vi "Simulation Angle Step (SubVI).vi"(6 "n":dbl, 7 "N (Rot)":u32, 8 "error in (no error)":errorcluster, 10 "Final Angle":dbl, 11 "VISA Refnum in":refnum<visa-resource-name>) -> (0 "error out":errorcluster, 2 "Next Angle":dbl, 3 "VISA Refnum out":refnum<visa-resource-name>, 4 "Angle Time Step (ms)":dbl, 5 "Rotation Complete?":bool)   [LabVIEW 2012]
uses:
  Stage Global.vi
  Rotation Mount Global.vi
panel:
  # "**For steps of the form degrees = a(x-xi)^n"
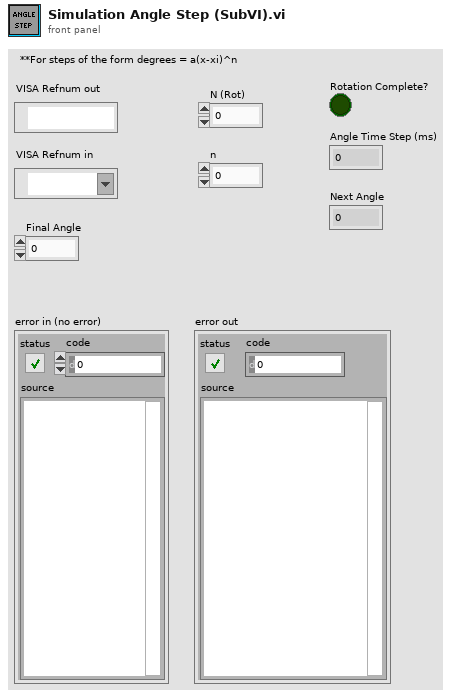
[diagram p1: front panel]
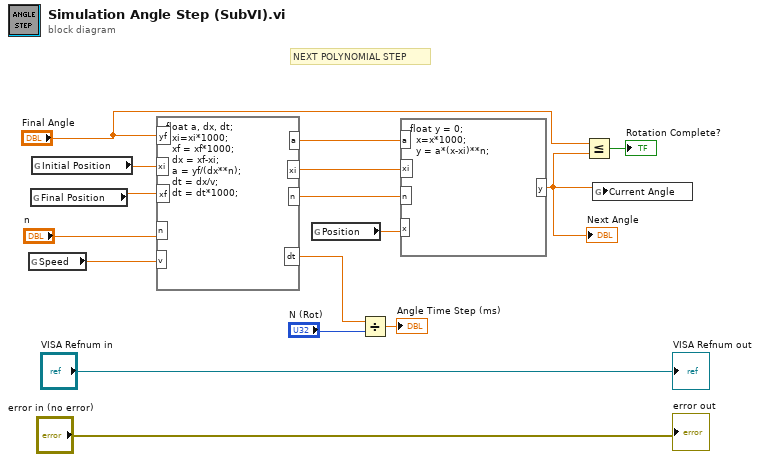
[diagram p0: block diagram]
diagram:
  # "NEXT POLYNOMIAL STEP"
  n1 = global read "Stage Global.vi" "Speed"() -> (w3:dbl)
  n2 = global read "Stage Global.vi" "Final Position"() -> (w8:dbl)
  n3 = global read "Stage Global.vi" "Initial Position"() -> (w9:dbl)
  n4 = formula code="float a, dx, dt;\n  xi=xi*1000;\n  xf = xf*1000;\n  dx = xf-xi;\n  a = yf/(dx**n);\n  dt = dx/v;\n  dt = dt*1000;"("xf"=w8, "xi"=w9, "yf"="Final Angle", "n"="n", "v"=w3) -> ("a"=w12:dbl, "xi"=w11:dbl, "n"=w10:dbl, "dt"=w2:dbl)
  n5 = global read "Stage Global.vi" "Position"() -> (w7:dbl)
  n6 = Divide(x=w2, y="N (Rot)") -> (x/y=→"Angle Time Step (ms)":dbl)
  n7 = formula code="float y = 0;\n  x=x*1000;\n  y = a*(x-xi)**n;"("a"=w12, "xi"=w11, "x"=w7, "n"=w10) -> ("y"=w6:dbl)
  "Next Angle" <- w6
  n8 = Less Or Equal?(x="Final Angle", y=w6) -> (x <= y?=→"Rotation Complete?":bool)
  n9 = global write "Rotation Mount Global.vi" "Current Angle"(w6) -> ()
  "VISA Refnum out" <- "VISA Refnum in"
  "error out" <- "error in (no error)"
